vi "TestVision_v3.vi"() -> ()   [LabVIEW 2019]
uses:
  <vilib>/vision/Pattern Matching.llb/IMAQ Curve Parameters.ctl
  <vilib>/vision/Shape Detection.llb/ShapeDetectionMatchOptions.ctl
  <vilib>/vision/Pattern Matching.llb/IMAQ Match Range Setting.ctl
  <vilib>/userDefined/High Color/IMAQdx.ctl
  <vilib>/vision/driver/NI_Vision_Acquisition_Software.lvlib
  <vilib>/vision/NI_Vision_Development_Module.lvlib
panel:
  out "CircleParams":string
  out "Image 3":T1(plugin-control)
  out "error out":errorcluster
  in  "Match Options":T2 {"Range Settings"."Match Constraints" items=["Rotation Angle (degrees)", "Scale Factor (%)", "Occlusion (%)"]}
  in  "Circle Descriptor":cluster{"Min Radius":dbl, "Max Radius":dbl}={"Min Radius"=90.0, "Max Radius"=500.0}
  out "Number of Matches Returned":i32
  out "Circles":T4(array[cluster]) {"Position"."Y" format="%.2f"; "Position"."X" format="%.2f"}
  in  "Curve Parameters":T5={"Extraction Mode"=0, "Edge Threshold"=100, "Edge Filter Size"=1, "Min Length"=10, "Row Search Step Size"=10, "Col Search Step Size"=100, "Max Endpoint Gap"=100, "Closed"=FALSE, "Subpixel"=FALSE} {"Max Endpoint Gap" min=0; "Col Search Step Size" min=1 max=255 step=1; "Row Search Step Size" min=1 max=255 step=1; "Min Length" min=0; "Edge Filter Size" items=["Fine", "Normal", "Controur Tracing"]; "Edge Threshold" min=1 max=65535 step=1; "Extraction Mode" items=["Normal", "Uniform Regions"]}
  in  "Image Type":T6 items=["Grayscale (U8)", "Grayscale (I16)", "Grayscale (SGL)", "Complex (CSG)", "RGB (U32)", "HSL (U32)", "RGB (U64)", "Grayscale (U16)"]
  # "Range"
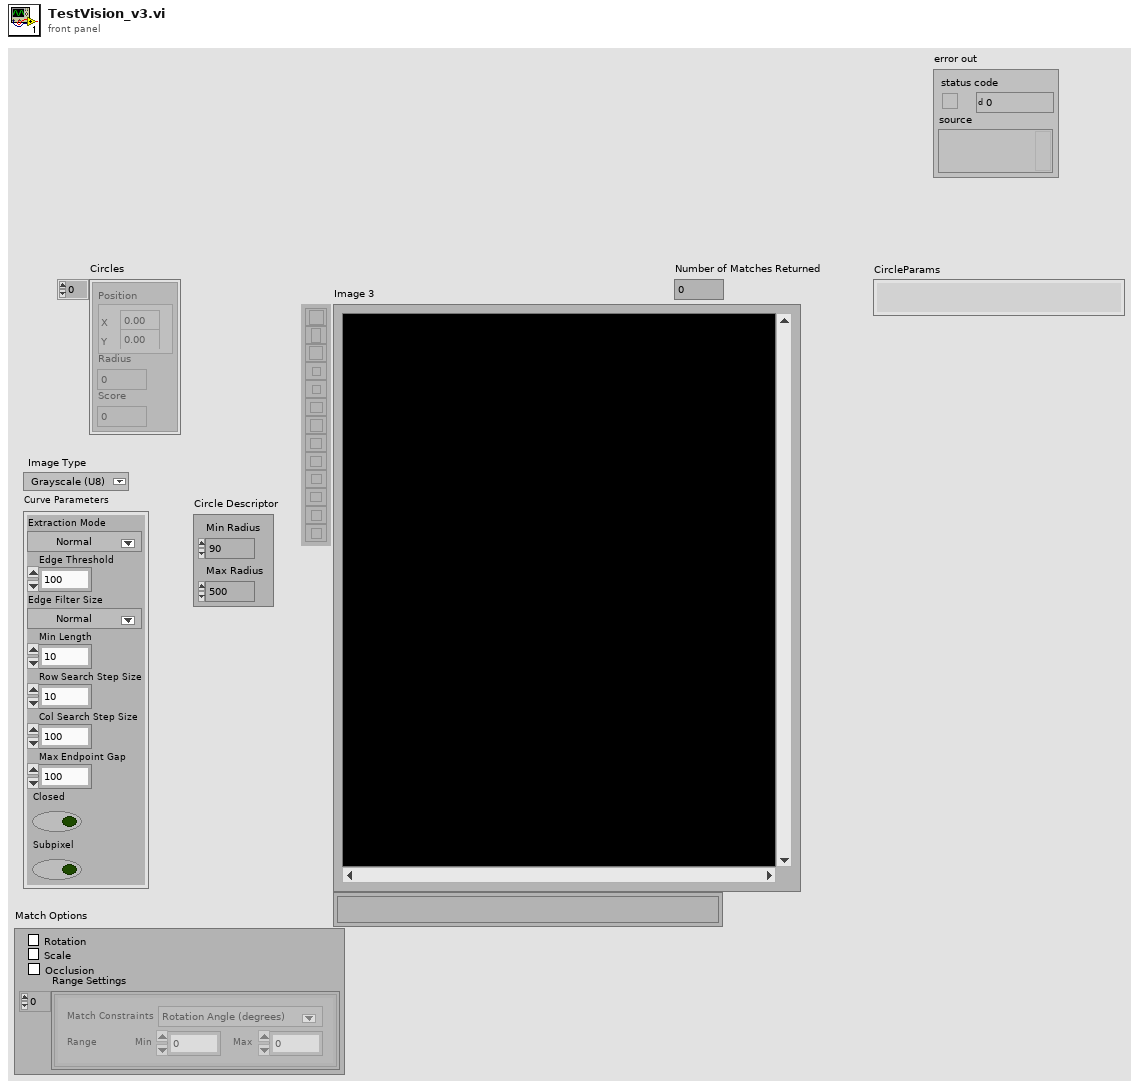
[diagram p1: front panel]
types:
  T1 = typedef "IMAQ Image.ctl" = refnum<image>
  T2 = typedef "ShapeDetectionMatchOptions.ctl" = cluster{"Rotation":bool, "Scale":bool, "Occlusion":bool, "Range Settings":T3[]}
  T3 = typedef "IMAQ Match Range Setting.ctl" = cluster{"Match Constraints":u32, "Min":dbl, "Max":dbl}
  T4 = cluster{"Position":cluster{"X":sgl, "Y":sgl}, "Radius":dbl, "Score":dbl}[]
  T5 = typedef "IMAQ Curve Parameters.ctl" = cluster{"Extraction Mode":u32, "Edge Threshold":i32, "Edge Filter Size":u32, "Min Length":i32, "Row Search Step Size":i32, "Col Search Step Size":i32, "Max Endpoint Gap":i32, "Closed":bool, "Subpixel":bool}
  T6 = typedef "Image Type" = u32
  T7 = typedef "IMAQ Circle" = cluster{"Center X":i32, "Center Y":i32, "Inner Radius":i32, "Outer Radius":i32, "Start Angle":dbl, "End Angle":dbl}
  T8 = typedef "IMAQdx.ctl" = refnum<k21>
  T9 = cluster{"Circles[0]":cluster{"Position":cluster{"X":sgl, "Y":sgl}, "Radius":dbl, "Score":dbl}, "Circles[1]":cluster{"Position":cluster{"X":sgl, "Y":sgl}, "Radius":dbl, "Score":dbl}, "Circles[2]":cluster{"Position":cluster{"X":sgl, "Y":sgl}, "Radius":dbl, "Score":dbl}, "Circles[3]":cluster{"Position":cluster{"X":sgl, "Y":sgl}, "Radius":dbl, "Score":dbl}, "Circles[4]":cluster{"Position":cluster{"X":sgl, "Y":sgl}, "Radius":dbl, "Score":dbl}, "Circles[5]":cluster{"Position":cluster{"X":sgl, "Y":sgl}, "Radius":dbl, "Score":dbl}, "Circles[6]":cluster{"Position":cluster{"X":sgl, "Y":sgl}, "Radius":dbl, "Score":dbl}, "Circles[7]":cluster{"Position":cluster{"X":sgl, "Y":sgl}, "Radius":dbl, "Score":dbl}, "Circles[8]":cluster{"Position":cluster{"X":sgl, "Y":sgl}, "Radius":dbl, "Score":dbl}}
  T10 = cluster{"Position":cluster{"X":sgl, "Y":sgl}, "Radius":dbl, "Score":dbl}
  T11 = typedef "ROI Descriptor" = cluster{"Global Rectangle":i32[], "Contours":cluster{"ID":enum32{"External", "Internal"}, "Type":u32, "Coordinates":i32[]}[]}
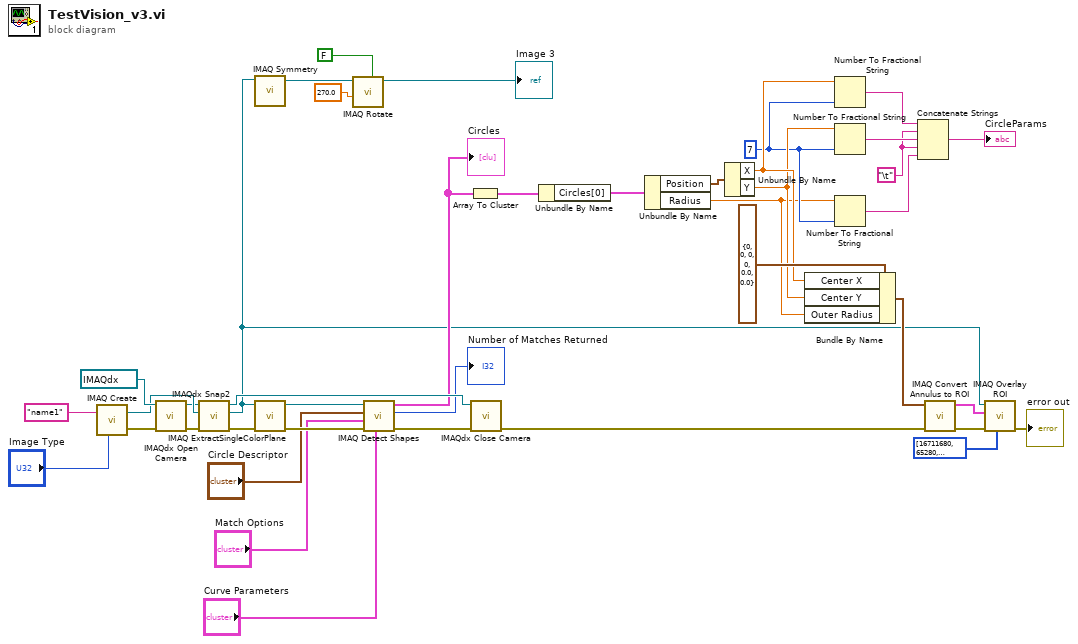
[diagram p0: block diagram]
diagram:
  w4 = "\t"
  w3 = i16 7 ("precision (6)")
  n1 = call "IMAQ Create"("Image Name"="name1", "Image Type"="Image Type") -> ("New Image"=w38:T1, "error out"=w35:errorcluster)  [unwired: 3 in]
  n2 = call <vilib>:"IMAQdx Open Camera.vi"("error in"=w35, "Session In"=T8 "cam0") -> ("error out"=w39:errorcluster, "Session Out"=w37:T8)  [unwired: 8 in]
  n3 = call <vilib>:"IMAQdx Snap2.vi"("error in"=w39, "Image In"=w38, "Session In"=w37) -> ("error out"=w31:errorcluster, "Image Out"=w10:T1, "Session Out"=w36:T8)  [unwired: 6 in]
  n4 = call "IMAQ Symmetry"("Image Src"=w10) -> ("Image Dst Out"=w14:T1)  [unwired: 4 in, 1 out]
  n5 = call "IMAQ ExtractSingleColorPlane"("error in (no error)"=w31, "Image Src"=w10) -> ("error out"=w30:errorcluster, "Image Dst Out"=w26:T1)  [unwired: 2 in, 6 out]
  n6 = call "IMAQ Rotate"("Maintain Size"=FALSE, "Angle (degrees)"=sgl 270.0, "Image Src"=w14) -> ("Image Dst Out"=→"Image 3":T1)  [unwired: 7 in, 1 out]
  n7 = call-poly "IMAQ Detect Shapes"("Curve Parameters"="Curve Parameters", "error in (no error)"=w30, "Match Options"="Match Options", "Circle Descriptor"="Circle Descriptor", "Image"=w26) -> ("error out"=w33:errorcluster, "Number of Matches Returned"=→"Number of Matches Returned":i32, "Circles"=w22:T4)  [unwired: 2 in, 2 out]
  "Circles" <- w22
  n8 = Array To Cluster(array=w22) -> (cluster=w21:T9)
  n9 = call <vilib>:"IMAQdx Close Camera.vi"("error in"=w33, "Session In"=w36) -> ("error out"=w19:errorcluster)  [unwired: 9 in]
  n10 = Unbundle By Name(w21) -> ("Circles[0]"=w20:T10)
  n11 = Unbundle By Name(w20) -> ("Position"=w23:cluster{"X":sgl, "Y":sgl}, "Radius"=w2:dbl)
  n12 = Unbundle By Name(w23) -> ("X"=w9:sgl, "Y"=w8:sgl)
  n13 = Bundle By Name(cluster=T7 {"Center X"=0, "Center Y"=0, "Inner Radius"=0, "Outer Radius"=0, "Start Angle"=0.0, "End Angle"=0.0} ("Annulus"), "Center X"=w9, "Center Y"=w8, "Outer Radius"=w2) -> (w25:T7)
  n14 = Number To Fractional String(number=w9, precision (6)=w3) -> (F-format string=w7:string)  [unwired: 2 in]
  n15 = Number To Fractional String(number=w8, precision (6)=w3) -> (F-format string=w6:string)  [unwired: 2 in]
  n16 = Number To Fractional String(number=w2, precision (6)=w3) -> (F-format string=w1:string)  [unwired: 2 in]
  n17 = Concatenate Strings(w7, w4, w6, w4, w1) -> (→"CircleParams":string)
  n18 = call "IMAQ Convert Annulus to ROI"("error in (no error)"=w19, "Annulus"=w25) -> ("error out"=w17:errorcluster, "ROI Descriptor"=w18:T11)  [unwired: 7 in]
  n19 = call "IMAQ Overlay ROI"("Colors (Green)"=u32[] [16711680, 65280, 2626303], "error in (no error)"=w17, "ROI Descriptor"=w18, "Image"=w10) -> ("error out"=→"error out":errorcluster)  [unwired: 6 in, 1 out]
